vi "InitEventStreamByIdAndCategory.vi"(8 "error in":errorcluster, 10 "Category":string, 11 "ID":string) -> (0 "error out":errorcluster, 3 "EventStreamInfo":T1)   [LabVIEW 2017]
uses:
  Types/SystemEventDataStruct.ctl
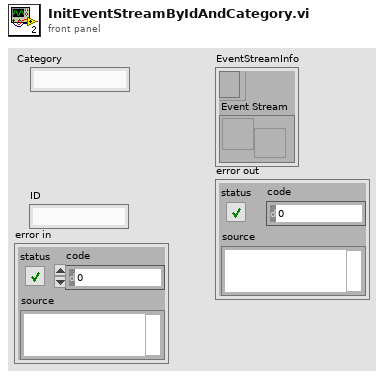
[diagram p1: front panel]
types:
  T1 = cluster{"Event Register":refnum<event-registration>, "Event Stream":refnum<user-event>}
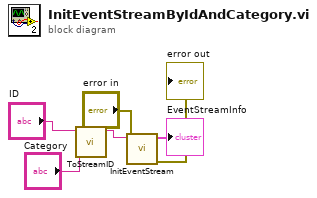
[diagram p0: block diagram]
diagram:
  n1 = call "ToStreamID.vi"("Category"="Category", "ID in"="ID") -> ("ID out"=w4:string)  [unwired: 9 in]
  n2 = call "InitEventStream.vi"("error in"="error in", "SteamID"=w4) -> ("error out"=→"error out":errorcluster, "EventStreamInfo"=→"EventStreamInfo":T1)  [unwired: 8 in]
